vi "Set Default.vi"(8 "error in (no error)":errorcluster, 11 "DMM Config Msg in":refnum<class "DMM Config Msg.lvclass">) -> (0 "error out":errorcluster, 3 "DMM Config Msg out":refnum<class "DMM Config Msg.lvclass">)   [LabVIEW 2020, in "DMM Msg.lvlib" / "DMM Config Msg.lvclass"]
doc: "Restore private data to a defined default state.\n\nThis implementation sets:\n10V DC with 6½ digits.\nAwait reply, -1ms timeout at normal priority without publish"
uses:
  DMM Config Msg.lvclass
  PPL/HDH.Driver.DMM.lvlibp/Controls/Ctl_Function.ctl
  PPL/HDH.Driver.DMM.lvlibp/Controls/Ctl_DigitResolution.ctl
  PPL/HDH.Actor Framework.Core.Actor.lvlibp/1abvi3w/vi.lib/ActorFramework/Message Enqueuer/Message Priority.ctl
  PPL/HDH.Actor Framework.Core.Publisher.lvlibp/Messages/Response Msg/Response Core/Controls/Ctl_SendFunction.ctl
  DMM Config Msg.lvclass/DMM Config Msg.ctl
  DMM Msg/DMM Msg.lvclass
  PPL/HDH.Driver.DMM.lvlibp
  PPL/HDH.Actor Framework.Core.Actor.lvlibp/1abvi3w/vi.lib/ActorFramework/Message Enqueuer/Message Enqueuer.lvclass
  PPL/HDH.Actor Framework.Core.Publisher.lvlibp
  PPL/HDH.Actor Framework.Core.Instrument Handler.lvlibp/Messages/Instrument Msg/Instrument Msg.lvclass
  C:/Current projects/WS/PPL/HDH.Actor Framework.Core.Instrument Handler.lvlibp/Messages/Instrument Msg/Instrument Msg.lvclass
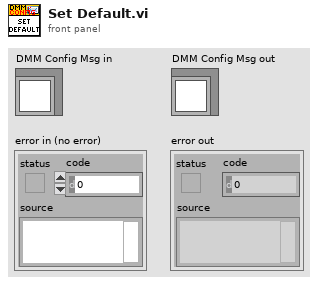
[diagram p1: front panel]
types:
  T1 = typedef "HDH.Actor Framework.Core.Publisher.lvlibp/Ctl_SendFunction.ctl" = enum16{"Send and Forget", "Request Reply", "Await Reply"}
  T2 = typedef "HDH.Actor Framework.Core.Actor.lvlibp/Message Enqueuer.lvclass/Message Priority.ctl" = enum16{"Low", "Normal", "High"}
  T3 = typedef "HDH.Driver.DMM.lvlibp/Ctl_DigitResolution.ctl" = enum8{"3½", "4½", "5½", "6½", "7½"}
  T4 = typedef "HDH.Driver.DMM.lvlibp/Ctl_Function.ctl" = enum8{"DC Volts", "AC Volts", "DC Current", "AC Current", "2-wire Resistance", "4-wire Resistance", "Diode", "Frequency", "Period", "AC Volts DC Coupled", "Capacitance", "Inductance", "Temperature"}
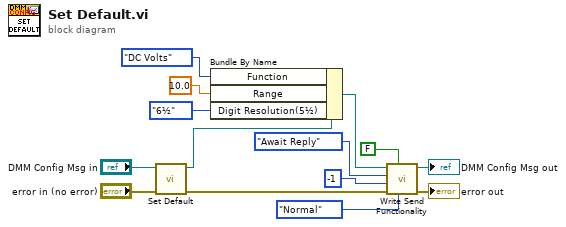
[diagram p0: block diagram]
diagram:
  n1 = call-parent "Set Default.vi"("error in (no error)"="error in (no error)", "Flex Msg in"="DMM Config Msg in") -> ("error out"=w5:errorcluster, "Flex Msg out"=w14:refnum<class "DMM Config Msg.lvclass">)  [unwired: 8 in]
  n2 = Bundle By Name(cluster=w14, "Function"=Ctl_Function."DC Volts", "Range"=10.0, "Digit Resolution(5½)"=Ctl_DigitResolution."6½") -> (w8:refnum<class "DMM Config Msg.lvclass">)
  n3 = call "Write Send Functionality.vi"("Message Priority(Normal)"=Message_Priority."Normal", "Publish Data?(T)"=FALSE, "error in (no error)"=w5, "Timeout if Waiting(-1ms)"=-1, "Send Function(Await Reply)"=Ctl_SendFunction."Await Reply", "Instrument Msg in"=w8) -> ("error out"=→"error out":errorcluster, "Instrument Msg out"=→"DMM Config Msg out":refnum<class "DMM Config Msg.lvclass">)  [unwired: 4 in]
